vi "PS_Discharge_Control.vi"(11 "On/Off":bool) -> (0 "error out":errorcluster)   [LabVIEW 2011]
uses:
  <vilib>/DAQmx/write.llb/DAQmx Write (Digital Bool 1Line 1Point).vi
  PS_Global.vi
  <vilib>/DAQmx/create/channels.llb/DAQmx Create Channel (DO-Digital Output).vi
  <vilib>/DAQmx/miscellaneous.llb/DAQmx Fill In Error Info.vi
panel:
  in  "USB Signal Generator?":bool=TRUE
  out "Read Back":string
  out "Check":string
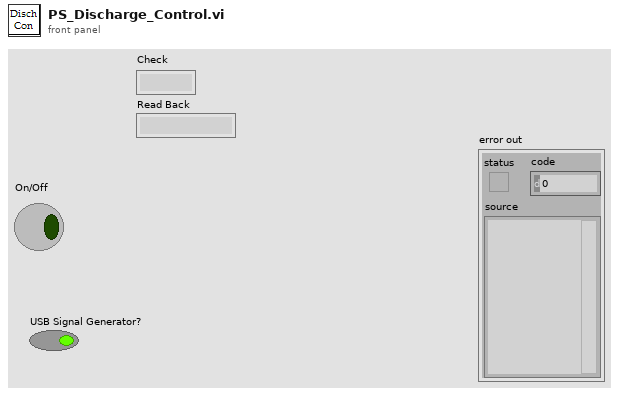
[diagram p1: front panel]
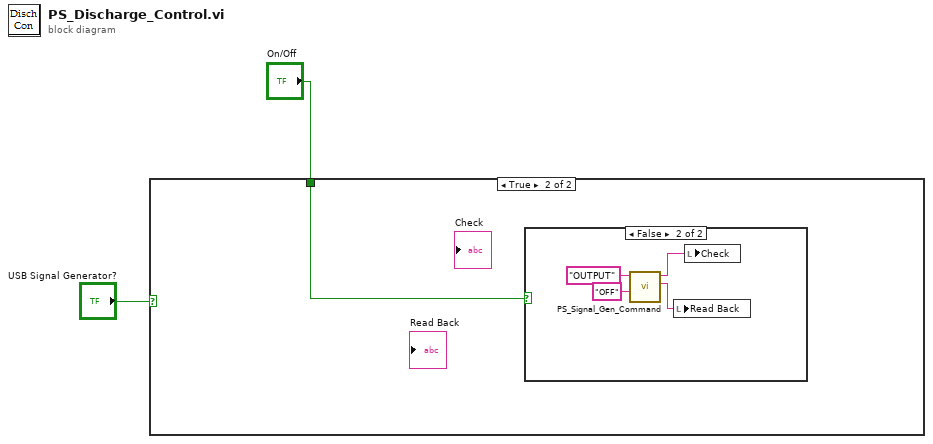
[diagram p0: block diagram]
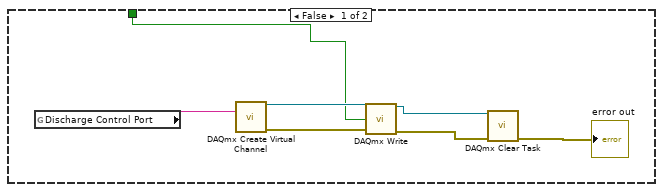
[diagram p2: hidden frame]
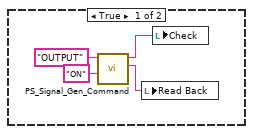
[diagram p3: hidden frame]
diagram:
  n1 = case shown="True" "USB Signal Generator?" {
    tunnel: "On/Off" -> [w7 w10]
    frame False {
      n2 = global read "PS_Global.vi" "Discharge Control Port"() -> (w9:tag)
      n3 = call-poly <vilib>:"DAQmx Create Virtual Channel.vi"("lines"=w9) -> ("task out"=w8:refnum<k21>, "error out"=w6:errorcluster)  [unwired: 13 in]
      n4 = call-poly <vilib>:"DAQmx Write.vi"("task/channels in"=w8, "data"=w7, "error in"=w6) -> ("task out"=w5:refnum<k21>, "error out"=w4:errorcluster)  [unwired: 10 in, 1 out]
      n5 = call <vilib>:"DAQmx Clear Task.vi"("task in"=w5, "error in"=w4) -> ("error out"=→"error out":errorcluster)  [unwired: 13 in]
    }
    frame True {
      n6 = case shown="False" w10 {
        frame True {
          n7 = call "PS_Signal_Gen_Command.vi"("Value String"="ON", "Command String"="OUTPUT") -> ("Read Back"=w14:string, "Request String"=w13:string)  [unwired: 7 in, 1 out]
          n8 = local write "Read Back"(w14) -> ()
          n9 = local write "Check"(w13) -> ()
        }
        frame False {
          n10 = call "PS_Signal_Gen_Command.vi"("Value String"="OFF", "Command String"="OUTPUT") -> ("Read Back"=w18:string, "Request String"=w17:string)  [unwired: 7 in, 1 out]
          n11 = local write "Read Back"(w18) -> ()
          n12 = local write "Check"(w17) -> ()
        }
      }
    }
  }
